vi "R(H)_VaryT_Runner.vi"() -> ()   [LabVIEW 2019]
uses:
  Components/Global 2.vi
  Components/DeltaRamp_globals.vi
  Components/B_Globals.vi
panel:
  out "Overall Progress":string="Step 7 of 11"
  out "Settle Progress":u8(slide) scale=0.0..100.0
  in  "Settle [Min]":dbl=5.0
  out "This Run":path=path "C:/User Data/gy251/20210406 EuS10-Cu (t)-EuS20/Delta_500uA_RH_T=16p00K.txt"
  out "Last Saved":path=path "C:/User Data/gy251/20210406 EuS10-Cu (t)-EuS20/Delta_500uA_RH_T=14p00K.txt"
  in  "Sample ID/Save Name":string="Delta_500uA_"
  in  "Save Directory":path=path "C:/User Data/gy251/20210406 EuS10-Cu (t)-EuS20"
  out "dT/dt SetP":dbl=0.5
  in  "Temp Rate [K/min]":dbl=0.5
  in  "Measure":bool
  out "dH/dt SetP":dbl=0.01
  out "Field SetP":dbl=0.05
  out "Temp SetP":dbl=16.0
  in  "Field [T] and Rate [T/min]":dbl[][](array[numeric])
  in  "Temps [K]":dbl[](array[numeric])
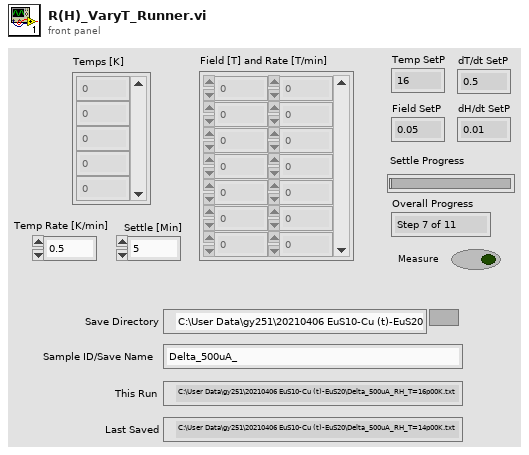
[diagram p1: front panel]
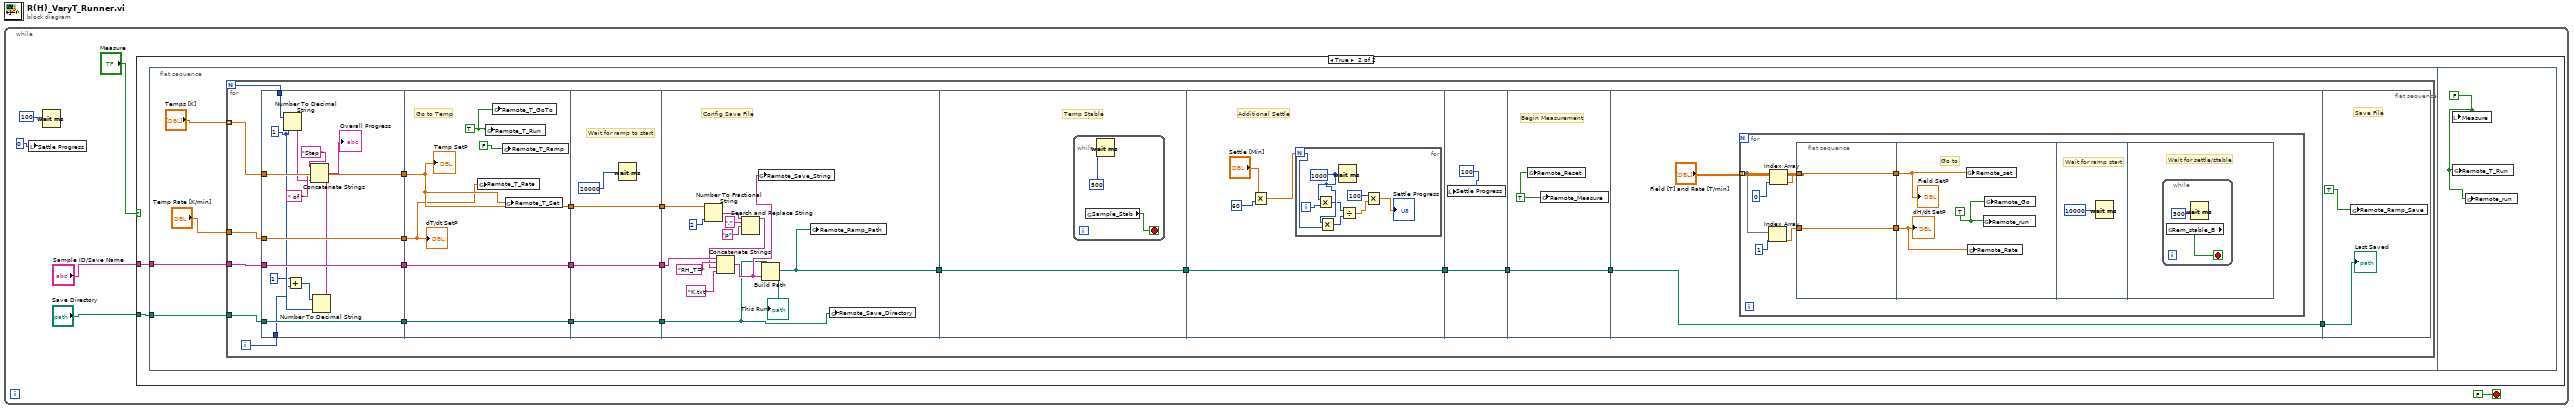
[diagram p0: block diagram]
diagram:
  n1 = while {
    stop <- FALSE stop-if-true
    n2 = local write "Settle Progress"(0) -> ()
    n3 = Wait (ms)(milliseconds to wait=100) -> ()  [unwired: 1 out]
    n4 = case shown="True" "Measure" {
      tunnel: "Sample ID/Save Name" -> [_ w8]
      tunnel: "Save Directory" -> [_ w7]
      frame False {
      }
      frame True {
        n5 = flat-sequence {
          tunnel: w8 -> [w10]
          tunnel: w7 -> [w9]
          frame #0 {
            n6 = for {
              N -> [w13]
              tunnel: "Temps [K]" -> [w34] mode=indexing
              tunnel: "Temp Rate [K/min]" -> [w33]
              tunnel: w10 -> [w32]
              tunnel: w9 -> [w31]
              i -> [w14]
              n7 = flat-sequence {
                tunnel: w31 -> [w45]
                tunnel: w32 -> [w46]
                tunnel: w33 -> [w47]
                tunnel: w34 -> [w48]
                tunnel: [w48] -> w18
                tunnel: [w47] -> w17
                tunnel: [w46] -> w16
                tunnel: [w45] -> w15
                tunnel: w14 -> [w36]
                tunnel: w13 -> [w44]
                tunnel: [w54] -> w24
                tunnel: [w53] -> w22
                tunnel: [w50] -> w20
                tunnel: w18 -> [w50]
                tunnel: w17 -> [w49]
                tunnel: w16 -> [w54]
                tunnel: w15 -> [w53]
                tunnel: w24 -> [w58]
                tunnel: [w58] -> w23
                tunnel: w22 -> [w57]
                tunnel: [w57] -> w21
                tunnel: w20 -> [w56]
                tunnel: [w56] -> w19
                tunnel: w23 -> [w70]
                tunnel: w21 -> [w60]
                tunnel: w19 -> [w66]
                tunnel: [w59] -> w27
                tunnel: [w71] -> w29
                tunnel: w27 -> [w71]
                tunnel: w29 -> [w77]
                tunnel: [w77] -> w28
                tunnel: w28 -> [w87]
                tunnel: [w87] -> w26
                tunnel: w26 -> [w89]
                tunnel: [w89] -> w25
                tunnel: [w90] -> w30
                tunnel: w25 -> [w90]
                tunnel: w30 -> [w108]
                frame #0 {
                  w43 = 1
                  n8 = Number To Decimal String(number=w44, width (-)=w43) -> (decimal integer string=w39:string)
                  n9 = Add(x=1, y=w36) -> (x+y=w35:i32)
                  n10 = Number To Decimal String(number=w35, width (-)=w43) -> (decimal integer string=w42:string)
                  n11 = Concatenate Strings("Step ", w42, " of ", w39) -> (→"Overall Progress":string)
                }
                frame #1 {
                  w52 = TRUE
                  # "Go to Temp"
                  n12 = global write "Global 2.vi" "Remote_T_Rate"(w49) -> ()
                  n13 = global write "Global 2.vi" "Remote_T_Run"(w52) -> ()
                  n14 = global write "Global 2.vi" "Remote_T_GoTo"(w52) -> ()
                  n15 = global write "Global 2.vi" "Remote_T_Ramp"(FALSE) -> ()
                  n16 = global write "Global 2.vi" "Remote_T_Set"(w50) -> ()
                  "Temp SetP" <- w50
                  "dT/dt SetP" <- w49
                }
                frame #2 {
                  # "Wait for ramp to start"
                  n17 = Wait (ms)(milliseconds to wait=20000) -> ()  [unwired: 1 out]
                }
                frame #3 {
                  # "Config Save File"
                  n18 = Number To Fractional String(number=w66, precision (6)=i16 2) -> (F-format string=w63:string)  [unwired: 2 in]
                  n19 = Search and Replace String(input string=w63, search string=".", replace string="p") -> (result string=w62:string)  [unwired: 5 in, 3 out]
                  n20 = Concatenate Strings(w70, "RH_T=", w62, "K.txt") -> (w61:string)
                  n21 = global write "DeltaRamp_globals.vi" "Remote_Save_String"(w61) -> ()
                  n22 = Build Path(base path=w60, name or relative path=w61) -> (appended path=w59:path)
                  "This Run" <- w59
                  n23 = global write "DeltaRamp_globals.vi" "Remote_Ramp_Path"(w59) -> ()
                  n24 = global write "DeltaRamp_globals.vi" "Remote_Save_Directory"(w60) -> ()
                }
                frame #4 {
                  # "Temp Stable"
                  n25 = while {
                    stop <- w73 stop-if-true
                    n26 = global read "Global 2.vi" "Sample_Stab"() -> (w73:bool)
                    n27 = Wait (ms)(milliseconds to wait=500) -> ()  [unwired: 1 out]
                  }
                }
                frame #5 {
                  # "Additional Settle"
                  n28 = Multiply(x="Settle [Min]", y=60) -> (x*y=w74:dbl)
                  n29 = for {
                    N: w74 -> [w84]
                    i -> [w85]
                    w83 = 1000
                    n30 = Multiply(x=w83, y=w85) -> (x*y=w81:i32)
                    n31 = Multiply(x=w83, y=w84) -> (x*y=w82:i32)
                    n32 = Wait (ms)(milliseconds to wait=w83) -> ()  [unwired: 1 out]
                    n33 = Divide(x=w81, y=w82) -> (x/y=w79:dbl)
                    n34 = Multiply(x=100, y=w79) -> (x*y=→"Settle Progress":dbl)
                  }
                }
                frame #6 {
                  n35 = local write "Settle Progress"(100) -> ()
                }
                frame #7 {
                  w88 = TRUE
                  # "Begin Measurement"
                  n36 = global write "DeltaRamp_globals.vi" "Remote_Reset"(w88) -> ()
                  n37 = global write "DeltaRamp_globals.vi" "Remote_Measure"(w88) -> ()
                }
                frame #8 {
                  n38 = for {
                    tunnel: "Field [T] and Rate [T/min]" -> [w96] mode=indexing
                    n39 = Index Array(array=w96, index=1) -> (element=w94:dbl)
                    n40 = Index Array(array=w96, index=0) -> (element=w97:dbl)
                    n41 = flat-sequence {
                      tunnel: w94 -> [w99]
                      tunnel: w97 -> [w100]
                      tunnel: [w100] -> w93
                      tunnel: [w99] -> w92
                      tunnel: w93 -> [w102]
                      tunnel: w92 -> [w101]
                      frame #0 {
                      }
                      frame #1 {
                        w103 = TRUE
                        # "Go to"
                        n42 = global write "B_Globals.vi" "Remote_set"(w102) -> ()
                        n43 = global write "B_Globals.vi" "Remote_Rate"(w101) -> ()
                        n44 = global write "B_Globals.vi" "Remote_run"(w103) -> ()
                        n45 = global write "B_Globals.vi" "Remote_Go"(w103) -> ()
                        "Field SetP" <- w102
                        "dH/dt SetP" <- w101
                      }
                      frame #2 {
                        # "Wait for ramp start"
                        n46 = Wait (ms)(milliseconds to wait=10000) -> ()  [unwired: 1 out]
                      }
                      frame #3 {
                        # "Wait for settle/stable"
                        n47 = while {
                          stop <- w105 stop-if-true
                          n48 = global read "B_Globals.vi" "Rem_stable_B"() -> (w105:bool)
                          n49 = Wait (ms)(milliseconds to wait=500) -> ()  [unwired: 1 out]
                        }
                      }
                    }
                  }
                }
                frame #9 {
                  # "Save File"
                  n50 = global write "DeltaRamp_globals.vi" "Remote_Ramp_Save"(TRUE) -> ()
                  "Last Saved" <- w108
                }
              }
            }
          }
          frame #1 {
            w109 = FALSE
            n51 = local write "Measure"(w109) -> ()
            n52 = global write "Global 2.vi" "Remote_T_Run"(w109) -> ()
            n53 = global write "B_Globals.vi" "Remote_run"(w109) -> ()
          }
        }
      }
    }
  }
